vi "Test_Process_Name.vi"(8 "error in (no error)":errorcluster, 10 "ProcessName":string, 11 "ProcessesList":string[](array[string])) -> (0 "error out":errorcluster, 2 "incorrectName":bool)   [LabVIEW 2011]
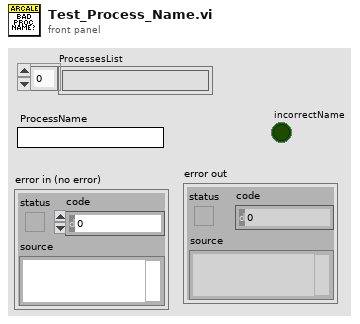
[diagram p1: front panel]
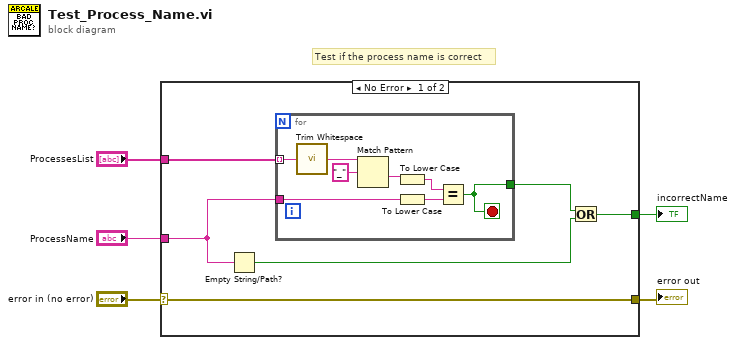
[diagram p0: block diagram]
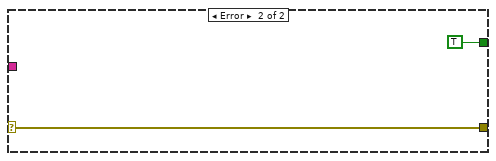
[diagram p2: hidden frame]
diagram:
  # "Test if the process name is correct"
  n1 = case shown="No Error" "error in (no error)" {
    selector: "error in (no error)" -> [w6 w20]
    tunnel: "ProcessName" -> [w10 _]
    tunnel: "ProcessesList" -> [w9 _]
    tunnel: [w8 TRUE] -> w3
    tunnel: [w6 w20] -> w1
    frame No Error {
      n2 = Empty String/Path?(string/path=w10) -> (empty?=w7:bool)
      n3 = for {
        tunnel: w9 -> [w18] mode=indexing
        tunnel: [w13] -> w11
        tunnel: w10 -> [w12]
        stop <- w13 stop-if-true
        n4 = call <vilib>:"Trim Whitespace.vi"("string"=w18) -> ("trimmed string"=w17:string)  [unwired: 1 in]
        n5 = Match Pattern(string=w17, regular expression="_") -> (after substring=w16:string)  [unwired: 1 in, 3 out]
        n6 = To Lower Case(string=w16) -> (all lower case string=w15:string)
        n7 = To Lower Case(string=w12) -> (all lower case string=w14:string)
        n8 = Equal?(x=w15, y=w14) -> (x = y?=w13:bool)
      }
      n9 = Or(x=w11, y=w7) -> (x .or. y?=w8:bool)
    }
    frame Error {
    }
  }
  "incorrectName" <- w3
  "error out" <- w1
